vi "SaveVseq.vi"(9 "ProjectName":string, 10 "ItemNames":string[][](array[string]), 11 "RootPath":path) -> (0 "error out":errorcluster)   [LabVIEW 2019]
uses:
  ROI/Controls/ROI_List_Action.ctl
  Caliper/Controls/Caliper_Entry_FGV_Action.ctl
  Coordinate/Control/CoordinateAction.ctl
  Controls/Parameter.ctl
  Controls/iVisionSEQ.ctl
  [Global]iVision_Version.vi
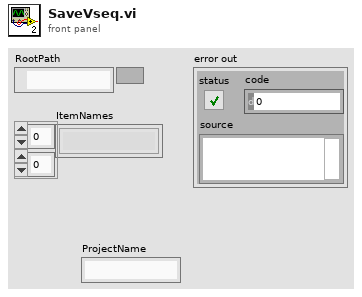
[diagram p1: front panel]
types:
  T1 = typedef "iVisionSEQ.ctl" = cluster{"iVision_Version":string, "iVisionSEQParam":variant}
  T2 = enum16{"Init", "Add", "Remove", "Read All", "Remove All", "WriteCriteria"}
  T3 = typedef "Caliper_Entry_FGV_Action.ctl" = enum16{"Init", "Close", "Add", "Delete", "ReplaceAll", "ReadAll"}
  T4 = typedef "Parameter.ctl" = enum16{"Initialize", "Write", "Read", "WriteAll", "Save", "Load"}
  T5 = typedef "CoordinateAction.ctl" = enum16{"Initialize", "CoordEntryInput", "CoordEntryOutput", "CoordEntryTemp", "CoordEntryBackup", "CoordEntryReturn"}
  T6 = enum16{"open", "replace", "create", "open or create", "replace or create", "replace or create with confirmation"}
  T7 = typedef "ROI_List_Action.ctl" = enum16{"Init", "Add ROI", "Delete ROI", "Get All ROI", "Get Specific ROI", "Set Analysis Setting", "Set Process Setting", "Replace All Entries", "ROIEntryBackup", "ROIEntryBackupClear", "ROIEntryReturn"}
  T8 = typedef "CoordinatteEntry.ctl" = cluster{"ProcessSetting":T9[], "Project Name":string, "AnalysisSetting":T11[], "Coord?":bool, "OriginPointInfo":cluster{"Output Original":bool, "Origin Name":string, "Angle":dbl, "Mode":u16, "OriginPoint":cluster{"X":dbl, "Y":dbl}}, "CaliperSetting":T13[], "CoordIndex":i32[]}
  T9 = typedef "Process_Setting.ctl" = cluster{"Enum_PreProcess":T10, "Parameter":string}
  T10 = typedef "VisionProcessName.ctl" = enum16{"*CamParameter*", "CamAttributes", "*Preprocess*", "CG_Brightness", "C_Plane Extraction", "C_Threshold", "G_Lookup Table", "G_Threshold"}
  T11 = typedef "CoordinateAnalysisSetting.ctl" = cluster{"Analysis_Type":enum16{"PatternMatch", "Straight Edge"}, "ROI ":T12, "Parameter":variant, "Step Result":variant, "AnalysisStepName":string, "CoordinateUse":bool}
  T12 = typedef "ROI Descriptor" = cluster{"Global Rectangle":i32[], "Contours":cluster{"ID":enum32{"External", "Internal"}, "Type":u32, "Coordinates":i32[]}[]}
  T13 = typedef "CoordinateCaliperSetting.ctl" = cluster{"Result":variant, "CoordinateUse":bool, "CaliperEntry":T14}
  T14 = typedef "CaliperDataEntry.ctl" = cluster{"CaliperType":T15, "Points":T16[], "Result":T18, "StepName":string}
  T15 = typedef "CaliperType.ctl" = u32
  T16 = typedef "SelectionListEntry.ctl" = cluster{"Type":T17, "Index":i32}
  T17 = typedef "SelectionListEntryPointType.ctl" = enum16{"AnalysisResult", "CaliperResult"}
  T18 = typedef "CaliperResult.ctl" = cluster{"PointInclude?":bool, "Num_Of_Pts":u8, "Position.X":dbl, "Position.Y":dbl, "Angle":dbl, "Distance":dbl, "Area":dbl, "Radius_MAX":dbl, "Radius2_min":dbl, "Dev_Residual":dbl, "P2.X":dbl, "P2.Y":dbl, "StepName":string, "Point ID":u8, "StepError?":bool, "ResultDiff?":bool}
  T19 = typedef "ParameterData.ctl" = cluster{"Rotate Angle":dbl, "Rotate?":bool, "Calibration File Path":string, "Cal?":bool}
  T20 = typedef "Vision_DataEntry.ctl" = cluster{"vROIName":string, "vROIContour":cluster{"Contour Type":u32, "ROI Type":u32, "Points":i32[]}, "ProcessSetting":T9[], "Analysis_Setting":T21}
  T21 = typedef "Analysis_Setting.ctl" = cluster{"PreProcess":T22, "Parameter":string}
  T22 = typedef "V_Analysis_Type.ctl" = enum16{"None", "C_Color Pattern Matching", "G_PatternMatching", "G_ShapeDectect", "G_GeometricMatch", "B_Area Check"}
  T23 = cluster{"OutputList":u16[], "Criteria Condition":string[]}
  T24 = cluster{"All ROI":T20[], "Output":cluster{"OutputList":u16[], "Criteria Condition":string[]}, string[][], "AllCaliperEntries":T14[], "CoordinatteEntry Output":T8, "ParameterData Out":T19, "AllCaliperEntries":T14[]}
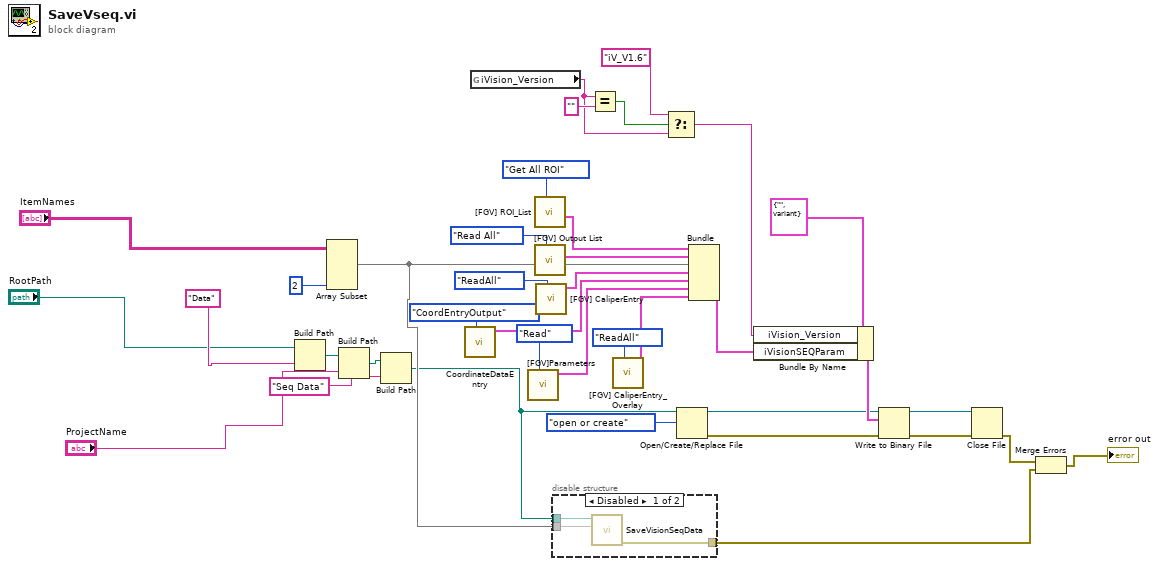
[diagram p0: block diagram]
diagram:
  n1 = Build Path(base path="RootPath", name or relative path="Data") -> (appended path=w23:path)
  n2 = Array Subset(array="ItemNames", length (col)=2 ("length")) -> (w35:string[][])  [unwired: 3 in]
  n3 = Build Path(base path=w23, name or relative path="ProjectName") -> (appended path=w16:path)
  n4 = Build Path(base path=w16, name or relative path="Seq Data") -> (appended path=w34:path)
  n5 = call "CoordinateDataEntry.vi"("CoordinateAction"=CoordinateAction."CoordEntryOutput") -> ("CoordinatteEntry Output"=w7:T8)  [unwired: 9 in, 1 out]
  n6 = global read "[Global]iVision_Version.vi" "iVision_Version"() -> (w3:string)
  n7 = call "[FGV]Parameters.vi"("Parameter"=Parameter."Read") -> ("ParameterData Out"=w26:T19)  [unwired: 9 in, 1 out]
  n8 = call "[FGV] ROI_List.vi"("Action"=ROI_List_Action."Get All ROI") -> ("All ROI"=w17:T20[])  [unwired: 8 in, 2 out]
  n9 = call "[FGV] Output List.vi"("Action"=T2."Read All") -> ("Output"=w29:T23)  [unwired: 9 in, 1 out]
  n10 = call "[FGV] CaliperEntry.vi"("Action"=Caliper_Entry_FGV_Action."ReadAll") -> ("AllCaliperEntries"=w9:T14[])  [unwired: 9 in, 1 out]
  n11 = disable-structure shown="Disabled" {
    disable-tunnel: [w41 _] -> w37
    disable-tunnel: w35 -> [w40 _]
    disable-tunnel: w34 -> [w39 _]
    frame Disabled {
      n12 = call "SaveVisionSeqData.vi"("AnalysisResult"=w40, "VisionSeqData"=w39) -> ("error out"=w41:errorcluster)  [unwired: 9 in]
    }
    frame Enabled {
    }
  }
  n13 = Equal?(x=w3, y="") -> (x = y?=w4:bool)
  n14 = call "[FGV] CaliperEntry_Overlay.vi"("Action"=Caliper_Entry_FGV_Action."ReadAll") -> ("AllCaliperEntries"=w28:T14[])  [unwired: 9 in, 1 out]
  n15 = Select(t="iV_V1.6", s=w4, f=w3) -> (s? t:f=w2:string)
  n16 = Open/Create/Replace File(file path (use dialog)=w34, operation (0:open)=T6."open or create") -> (refnum out=w22:refnum<file>, error out=w20:errorcluster)  [unwired: 4 in, 1 out]
  n17 = Bundle("All ROI"=w17, "Output"=w29, w35, "AllCaliperEntries"=w9, "CoordinatteEntry Output"=w7, "ParameterData Out"=w26, "AllCaliperEntries"=w28) -> (w32:T24)  [unwired: 1 in]
  n18 = Bundle By Name(cluster=T1 {"iVision_Version"="", "iVisionSEQParam"=variant} ("iVisionSEQ"), "iVision_Version"=w2, "iVisionSEQParam"=w32) -> (w33:T1)
  n19 = Write to Binary File(file (use dialog)=w22, data=w33, error in=w20) -> (refnum out=w21:refnum<file>, error out=w19:errorcluster)  [unwired: 3 in, 1 out]
  n20 = Close File(refnum=w21, error in=w19) -> (error out=w36:errorcluster)  [unwired: 1 out]
  n21 = Merge Errors(w36, w37) -> (→"error out":errorcluster)
